vi "Run Bfr Tx - Sim Buffer Data.vi"(8 "error in (no error)":errorcluster, 11 "Tx Loop Data in":T1={"General Resources"={"Packet Name"="", "Packet ID"=0, "Local IP Address"="", "Local Port"=0, "Multicast"=FALSE, "Multicast IP Address"=0, "Header Info"=[], "Byte Order"=enum."big-endian, network order", "Channel Data Types"=[], "Duplex Packets"=refnum}, "Header Details"={"Packet Size"=0, "Protocol Revision"=0, "System Definition Version"=0, "Source Node Name"="", "Packet ID"=0, "Number of Channels"=0, "Static Header Size"=0, "Total Header Size"=0, "CustomHeaderLogic"={"CustomHeaderON"=FALSE, "CustomHeaderLogic"=""}}, "Buffer Resources"={"Data Buffer"=0, "Pointer Encoding"=enum."Direct Encoding", "Buffer Size"=0, "Buffer Size (I32)"=0, "Raw Buffer Data"=[], "Is Buffered"=FALSE, "External Buffer"=FALSE, "Prepend Header"=FALSE, "Valid Buffer"=FALSE}, "Runtime Resources"={"Connection ID"=refnum, "Transmit Option"=enum."Always", "Destination IP Address"=0, "Destination Port"=0, "Multicast IP Address"=0, "TTL"=0, "Multicast"=FALSE, "Port as Channel"=FALSE, "ExecutionConfig"={"Loop Period"=0, "RT Loop Period"=-2, "Untimed Period"=0, "Target Processor"=0, "Priority"=0, "Thread Management"=enum."Untimed (Default)"}}, "Echo Resources"={"Transmit Echo Option"=enum."PCL Reset", "Packet Count"=0.0, "Counter Increment"=0.0, "Transmit Values"=[]}, "Buffer Option Support"={"Buffer Option"=enum."Static Buffer", "Sim Option"=enum."No Simulation"}, "Channel Resources"={"Transmit Flag"=refnum, "Transmit Echo"=refnum, "Transmit Bytes"=refnum, "Port Channel"=refnum, "Buffer (External)"=refnum, "Buffer (Local)"=refnum, "Timestamp"=refnum}, "Debug Resources"={"Debug Mode"=FALSE, "Debug Log File"=refnum, "Packet Name"=""}} {"Buffer Resources"."Data Buffer" format="%016x"}) -> (0 "error out":errorcluster, 3 "Tx Loop Data out":T1={"General Resources"={"Packet Name"="", "Packet ID"=0, "Local IP Address"="", "Local Port"=0, "Multicast"=FALSE, "Multicast IP Address"=0, "Header Info"=[], "Byte Order"=enum."big-endian, network order", "Channel Data Types"=[], "Duplex Packets"=refnum}, "Header Details"={"Packet Size"=0, "Protocol Revision"=0, "System Definition Version"=0, "Source Node Name"="", "Packet ID"=0, "Number of Channels"=0, "Static Header Size"=0, "Total Header Size"=0, "CustomHeaderLogic"={"CustomHeaderON"=FALSE, "CustomHeaderLogic"=""}}, "Buffer Resources"={"Data Buffer"=0, "Pointer Encoding"=enum."Direct Encoding", "Buffer Size"=0, "Buffer Size (I32)"=0, "Raw Buffer Data"=[], "Is Buffered"=FALSE, "External Buffer"=FALSE, "Prepend Header"=FALSE, "Valid Buffer"=FALSE}, "Runtime Resources"={"Connection ID"=refnum, "Transmit Option"=enum."Always", "Destination IP Address"=0, "Destination Port"=0, "Multicast IP Address"=0, "TTL"=0, "Multicast"=FALSE, "Port as Channel"=FALSE, "ExecutionConfig"={"Loop Period"=0, "RT Loop Period"=-2, "Untimed Period"=0, "Target Processor"=0, "Priority"=0, "Thread Management"=enum."Untimed (Default)"}}, "Echo Resources"={"Transmit Echo Option"=enum."PCL Reset", "Packet Count"=0.0, "Counter Increment"=0.0, "Transmit Values"=[]}, "Buffer Option Support"={"Buffer Option"=enum."Static Buffer", "Sim Option"=enum."No Simulation"}, "Channel Resources"={"Transmit Flag"=refnum, "Transmit Echo"=refnum, "Transmit Bytes"=refnum, "Port Channel"=refnum, "Buffer (External)"=refnum, "Buffer (Local)"=refnum, "Timestamp"=refnum}, "Debug Resources"={"Debug Mode"=FALSE, "Debug Log File"=refnum, "Packet Name"=""}} {"Buffer Resources"."Data Buffer" format="%016x"})   [LabVIEW 2019, in "UDP-Custom-Device Engine.lvlib"]
uses:
  UDP-Custom-Device Engine.lvlib
  Types/Engine - Buffered Tx Loop Data.ctl
  Types/Engine - General Resources.ctl
  <vilib>/NI VeriStand/VeriStand Data/Typedefs/Typedefs.Data Types.ctl
  Shared/Types/Shared - Duplex Settings.ctl
  Shared/Types/Shared - Header Details.ctl
  Shared/Types/Shared - Custom Header.ctl
  Types/Engine - Buffer Resources.ctl
  Shared/Types/Shared - Pointer Encoding.ctl
  Types/Engine - Tx Runtime Resources.ctl
  Shared/Types/Shared - Transmit Flag Options.ctl
  Types/Engine - Execution Config.ctl
  Shared/Types/Shared - Thread Management.ctl
  Types/Engine - Tx Echo Resources.ctl
  Shared/Types/Shared - Transmit Echo Options.ctl
  Types/Engine - Buffered Tx Buffer Option Support.ctl
  Shared/Types/Shared - Transmit Buffer Options.ctl
  Shared/Types/Shared - Transmit Sim Options.ctl
  Types/Engine - Buffered Tx Channel Refs.ctl
  <vilib>/NI/NIVS Inline Async API/_Data Access Engine/Data Access Engine/Types/Read.DVR.ctl
  <vilib>/NI/NIVS Inline Async API/_Data Access Engine/Access Type Classes/Read/Read.lvclass
  <vilib>/NI/NIVS Inline Async API/_Data Access Engine/Data Access Engine/Types/Write.DVR.ctl
  <vilib>/NI/NIVS Inline Async API/_Data Access Engine/Access Type Classes/Write/Write.lvclass
  Types/Engine - Debug Resources.ctl
  <vilib>/NI/NIVS Inline Async API/_Data Access Engine/Access Type Classes/Read/Read.lvclass/Read.ctl
  <vilib>/NI VeriStand/VeriStand Data/Pointer Operations/Pointer.Write (String).vi
  <vilib>/NI VeriStand/VeriStand Data/Pointer Operations/Pointer.Write (1D U8).vi
  <vilib>/NI VeriStand/VeriStand Data/Pointer Operations/Pointer.Write (I32).vi
  <vilib>/NI VeriStand/VeriStand Data/Pointer Operations/Pointer.Write (U16).vi
  Transmit/Run Tx - Handle Transmit Option.vi
  Run Bfr Tx - Handle Transmit Size.vi
  Transmit/Run Tx - Handle Port Tx Check.vi
  <vilib>/NI/NIVS Inline Async API/_Data Access Engine/Data Access Engine/Methods/Data.Processes.Execute.vi
  <vilib>/NI/NIVS Inline Async API/_Data Access Engine/Data Access Engine/Methods/Read.Data.vi
  <vilib>/NI VeriStand/VeriStand Data/Type Conversion/Type Conversion.From Double.vi
  <vilib>/NI VeriStand/VeriStand Data/Type Conversion/Type Conversion.From Double (I32).vi
  <vilib>/NI/NIVS Inline Async API/_Data Access Engine/Access Type Classes/Read/Read.ProcessData.vi
  <vilib>/NI VeriStand/VeriStand Data/VeriStand Data.lvlib
  Shared/UDP-Custom-Device Shared.lvlib
  <vilib>/NI/NIVS Inline Async API/_Data Access Engine/Data Access Engine/Data Access Engine.lvclass
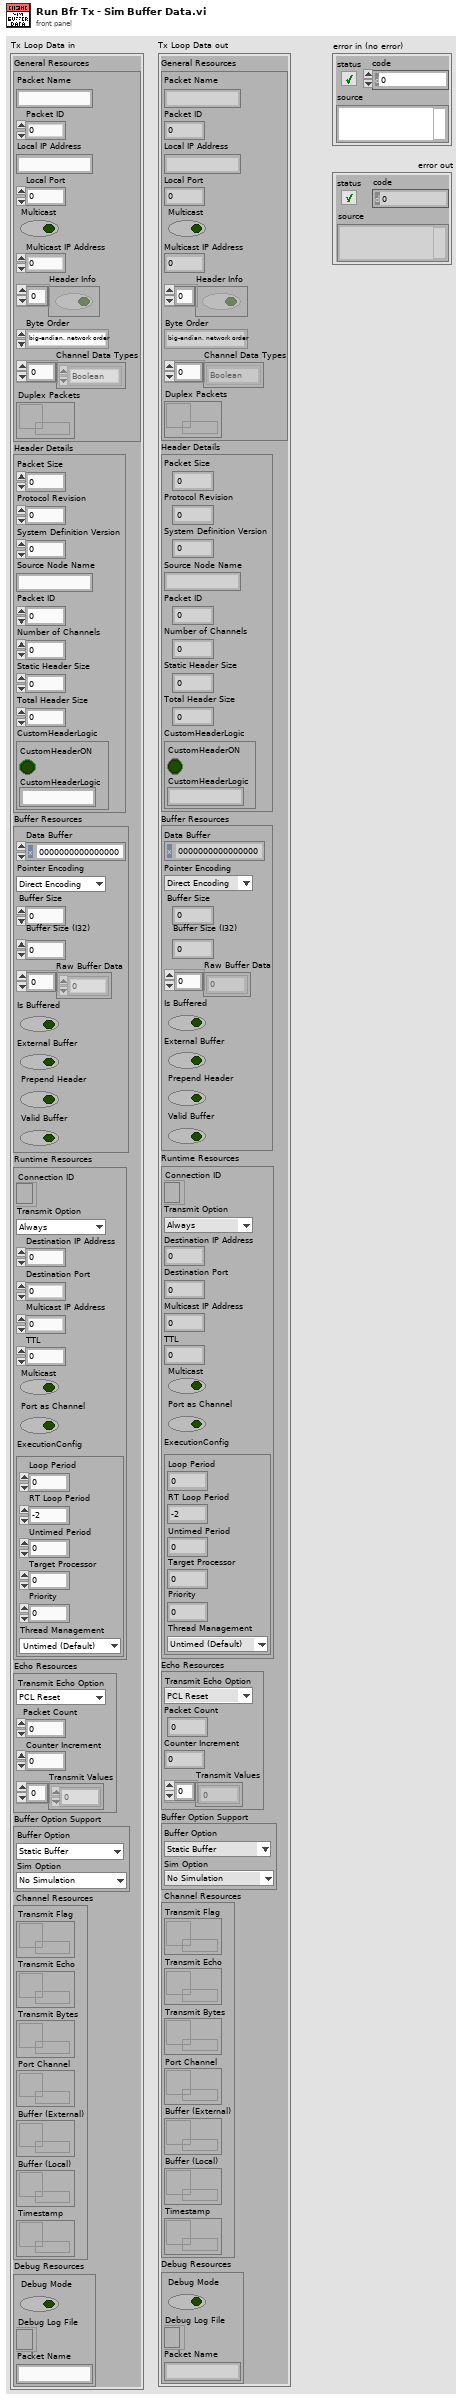
[diagram p1: front panel]
types:
  T1 = typedef "UDP-Custom-Device Engine.lvlib/Engine - Buffered Tx Loop Data.ctl" = cluster{"General Resources":T2, "Header Details":T4, "Buffer Resources":T6, "Runtime Resources":T8, "Echo Resources":T12, "Buffer Option Support":T14, "Channel Resources":T17, "Debug Resources":T20}
  T2 = typedef "UDP-Custom-Device Engine.lvlib/Engine - General Resources.ctl" = cluster{"Packet Name":string, "Packet ID":i32, "Local IP Address":string, "Local Port":i32, "Multicast":bool, "Multicast IP Address":u32, "Header Info":bool[], "Byte Order":enum16{"big-endian, network order", "native, host order", "little-endian"}, "Channel Data Types":T3[], "Duplex Packets":refnum<data-value>}
  T3 = typedef "VeriStand Data.lvlib/Typedefs.Data Types.ctl" = enum16{"Boolean", "Single", "Double", "I8", "I16", "I32", "I64", "U8", "U16", "U32", "U64"}
  T4 = typedef "UDP-Custom-Device Shared.lvlib/Shared - Header Details.ctl" = cluster{"Packet Size":u16, "Protocol Revision":u8, "System Definition Version":u64, "Source Node Name":string, "Packet ID":u32, "Number of Channels":u32, "Static Header Size":u16, "Total Header Size":u16, "CustomHeaderLogic":T5}
  T5 = typedef "UDP-Custom-Device Shared.lvlib/Shared - Custom Header.ctl" = cluster{"CustomHeaderON":bool, "CustomHeaderLogic":string}
  T6 = typedef "UDP-Custom-Device Engine.lvlib/Engine - Buffer Resources.ctl" = cluster{"Data Buffer":u64, "Pointer Encoding":T7, "Buffer Size":u64, "Buffer Size (I32)":i32, "Raw Buffer Data":u8[], "Is Buffered":bool, "External Buffer":bool, "Prepend Header":bool, "Valid Buffer":bool}
  T7 = typedef "UDP-Custom-Device Shared.lvlib/Shared - Pointer Encoding.ctl" = enum16{"Direct Encoding", "Conversion Encoding"}
  T8 = typedef "UDP-Custom-Device Engine.lvlib/Engine - Tx Runtime Resources.ctl" = cluster{"Connection ID":refnum<k16>, "Transmit Option":T9, "Destination IP Address":u32, "Destination Port":u16, "Multicast IP Address":u32, "TTL":u16, "Multicast":bool, "Port as Channel":bool, "ExecutionConfig":T10}
  T9 = typedef "UDP-Custom-Device Shared.lvlib/Shared - Transmit Flag Options.ctl" = enum16{"Always", "One-Shot", "Toggle"}
  T10 = typedef "UDP-Custom-Device Engine.lvlib/Engine - Execution Config.ctl" = cluster{"Loop Period":i64, "RT Loop Period":i64, "Untimed Period":u32, "Target Processor":i32, "Priority":i32, "Thread Management":T11}
  T11 = typedef "UDP-Custom-Device Shared.lvlib/Shared - Thread Management.ctl" = enum16{"Untimed (Default)", "Timed (High Priority)"}
  T12 = typedef "UDP-Custom-Device Engine.lvlib/Engine - Tx Echo Resources.ctl" = cluster{"Transmit Echo Option":T13, "Packet Count":dbl, "Counter Increment":dbl, "Transmit Values":dbl[]}
  T13 = typedef "UDP-Custom-Device Shared.lvlib/Shared - Transmit Echo Options.ctl" = enum16{"PCL Reset", "Counter", "Mirror"}
  T14 = typedef "UDP-Custom-Device Engine.lvlib/Engine - Buffered Tx Buffer Option Support.ctl" = cluster{"Buffer Option":T15, "Sim Option":T16}
  T15 = typedef "UDP-Custom-Device Shared.lvlib/Shared - Transmit Buffer Options.ctl" = enum16{"Static Buffer", "FIFO Buffer", "FIFO Buffer + Port"}
  T16 = typedef "UDP-Custom-Device Shared.lvlib/Shared - Transmit Sim Options.ctl" = enum16{"No Simulation", "Counter", "Full Buffer", "FIFO Test", "FIFO + Port Test"}
  T17 = typedef "UDP-Custom-Device Engine.lvlib/Engine - Buffered Tx Channel Refs.ctl" = cluster{"Transmit Flag":T18, "Transmit Echo":T19, "Transmit Bytes":T18, "Port Channel":T18, "Buffer (External)":T18, "Buffer (Local)":T19, "Timestamp":T18}
  T18 = typedef "Data Access Engine.lvlib/Data Access Engine.lvclass/Read.DVR.ctl" = refnum<data-value>
  T19 = typedef "Data Access Engine.lvlib/Data Access Engine.lvclass/Write.DVR.ctl" = refnum<data-value>
  T20 = typedef "UDP-Custom-Device Engine.lvlib/Engine - Debug Resources.ctl" = cluster{"Debug Mode":bool, "Debug Log File":refnum<file>, "Packet Name":string}
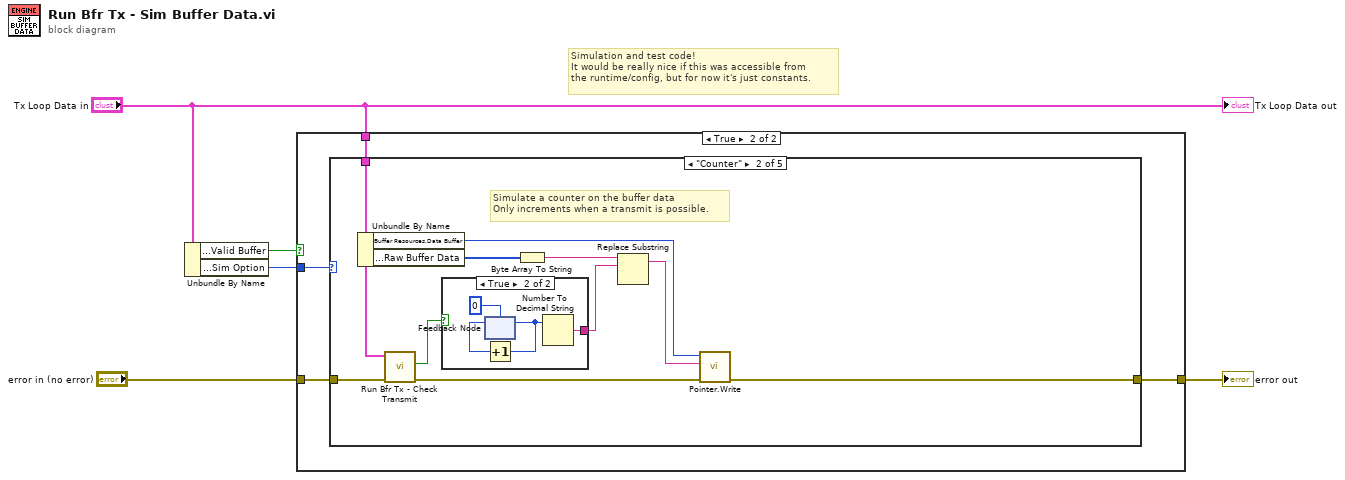
[diagram p0: block diagram]
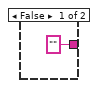
[diagram p4: hidden frame]
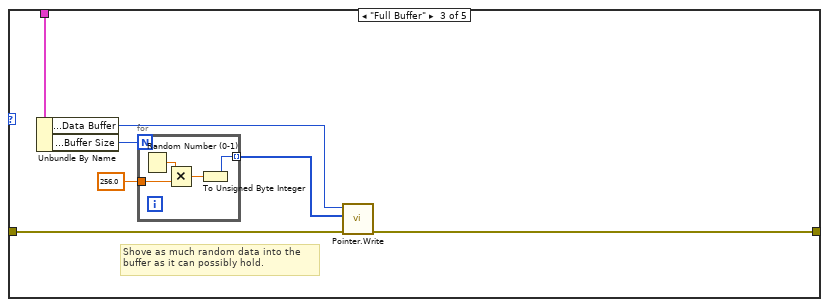
[diagram p5: hidden frame]
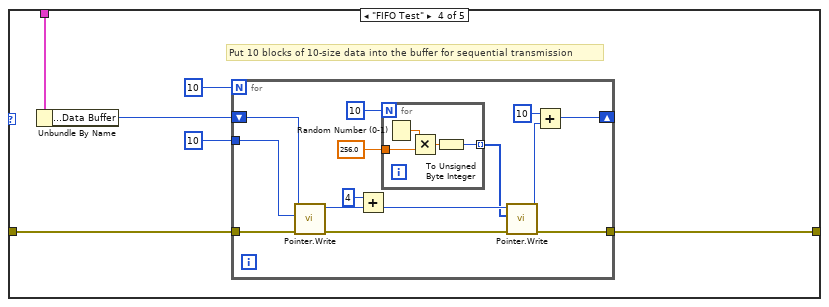
[diagram p6: hidden frame]
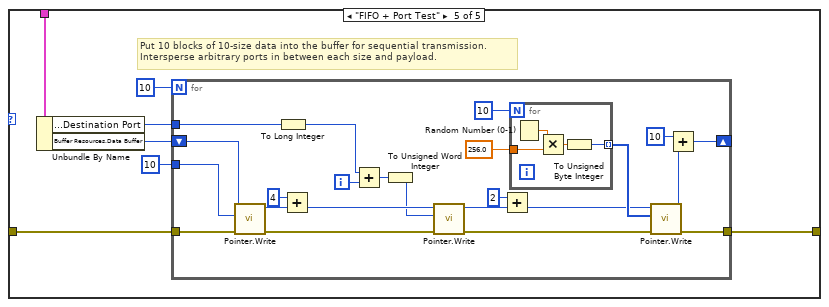
[diagram p7: hidden frame]
diagram:
  # "Simulation and test code!\nIt would be really nice if this was accessible from\nthe runtime/config, but for now it's just constants."
  n1 = Unbundle By Name("Tx Loop Data in") -> ("Buffer Resources.Valid Buffer"=w2:bool, "Buffer Option Support.Sim Option"=w1:T16)
  n2 = case shown="True" w2 {
    tunnel: "error in (no error)" -> [w6 w10]
    tunnel: [w6 w9] -> w4
    tunnel: "Tx Loop Data in" -> [_ w8]
    tunnel: w1 -> [_ w7]
    frame False {
    }
    frame True {
      n3 = case shown="\"Counter\"" w7 {
        tunnel: w8 -> [_ w15 w33 w43 w68]
        tunnel: w10 -> [w11 w14 w31 w39 w64]
        tunnel: [w11 w19 w30 w41 w66] -> w9
        frame "No Simulation", Default {
          # "No simulation data in normal\nbehavior."
        }
        frame "Counter" {
          # "Simulate a counter on the buffer data\nOnly increments when a transmit is possible."
          n4 = Unbundle By Name(w15) -> ("Buffer Resources.Data Buffer"=w21:u64, "Buffer Resources.Raw Buffer Data"=w17:u8[])
          n5 = call "Run Bfr Tx - Check Transmit.vi"("error in (no error)"=w14, "Tx Loop Data in"=w15) -> ("error out"=w13:errorcluster, "Transmit?"=w12:bool)  [unwired: 6 in, 2 out]
          n6 = case shown="True" w12 {
            tunnel: ["" w23] -> w20
            frame False {
            }
            frame True {
              n7 = feedback #1(0) -> (w25:i32)
              n8 = Increment(x=w25) -> (x+1=w24:i32)
              n9 = feedback-in #1(w24) -> ()
              n10 = Number To Decimal String(number=w24) -> (decimal integer string=w23:string)  [unwired: 1 in]
            }
          }
          n11 = Byte Array To String(unsigned byte array=w17) -> (string=w16:string)
          n12 = Replace Substring(4:w20, 5:w16) -> (1:w18:string)  [unwired: 2 in, 1 out]
          n13 = call-poly <vilib>:"Pointer.Write.vi"("error in (no error)"=w13, "string in"=w18, "pointer in"=w21) -> ("error out"=w19:errorcluster)  [unwired: 6 in, 2 out]
        }
        frame "Full Buffer" {
          # "Shove as much random data into the\nbuffer as it can possibly hold."
          n14 = Unbundle By Name(w33) -> ("Buffer Resources.Data Buffer"=w32:u64, "Buffer Resources.Buffer Size"=w29:u64)
          n15 = for {
            N: w29 -> [_]
            tunnel: [w34] -> w27 mode=indexing
            tunnel: 256.0 -> [w36]
            n16 = Random Number (0-1)() -> (number: 0 to 1=w37:dbl)
            n17 = Multiply(x=w37, y=w36) -> (x*y=w35:dbl)
            n18 = To Unsigned Byte Integer(number=w35) -> (unsigned 8bit integer=w34:u8)
          }
          n19 = call-poly <vilib>:"Pointer.Write.vi"("error in (no error)"=w31, "values"=w27, "pointer in"=w32) -> ("error out"=w30:errorcluster)  [unwired: 6 in, 2 out]
        }
        frame "FIFO Test" {
          # "Put 10 blocks of 10-size data into the buffer for sequential transmission"
          n20 = Unbundle By Name(w43) -> ("Buffer Resources.Data Buffer"=w42:u64)
          n21 = for {
            N: 10 -> [_]
            tunnel: [w57] -> w41
            tunnel: w39 -> [w55]
            tunnel: 10 -> [w53]
            shift-right: [w44] -> _
            shift-left: w42 -> [w56]
            n22 = call-poly <vilib>:"Pointer.Write.vi"("error in (no error)"=w55, "value"=w53, "pointer in"=w56) -> ("error out"=w54:errorcluster, "pointer out"=w51:u64)  [unwired: 6 in, 1 out]
            n23 = Add(x=u64 4, y=w51) -> (x+y=w50:u64)
            n24 = for {
              N: 10 -> [_]
              tunnel: [w58] -> w47 mode=indexing
              tunnel: 256.0 -> [w60]
              n25 = Random Number (0-1)() -> (number: 0 to 1=w61:dbl)
              n26 = Multiply(x=w61, y=w60) -> (x*y=w59:dbl)
              n27 = To Unsigned Byte Integer(number=w59) -> (unsigned 8bit integer=w58:u8)
            }
            n28 = call-poly <vilib>:"Pointer.Write.vi"("error in (no error)"=w54, "values"=w47, "pointer in"=w50) -> ("error out"=w57:errorcluster, "pointer out"=w45:u64)  [unwired: 6 in, 1 out]
            n29 = Add(x=u64 10, y=w45) -> (x+y=w44:u64)
          }
        }
        frame "FIFO + Port Test" {
          # "Put 10 blocks of 10-size data into the buffer for sequential transmission.\nIntersperse arbitrary ports in between each size and payload."
          n30 = Unbundle By Name(w68) -> ("Runtime Resources.Destination Port"=w62:u16, "Buffer Resources.Data Buffer"=w67:u64)
          n31 = for {
            N: 10 -> [_]
            tunnel: [w91] -> w66
            tunnel: w64 -> [w89]
            tunnel: 10 -> [w88]
            shift-right: [w80] -> _
            shift-left: w67 -> [w90]
            tunnel: w62 -> [w70]
            i -> [w72]
            n32 = call-poly <vilib>:"Pointer.Write.vi"("error in (no error)"=w89, "value"=w88, "pointer in"=w90) -> ("error out"=w78:errorcluster, "pointer out"=w86:u64)  [unwired: 6 in, 1 out]
            n33 = To Long Integer(number=w70) -> (32bit integer=w69:i32)
            n34 = Add(x=u64 4, y=w86) -> (x+y=w79:u64)
            n35 = Add(x=w69, y=w72) -> (x+y=w73:i32)
            n36 = To Unsigned Word Integer(number=w73) -> (unsigned 16bit integer=w71:u16)
            n37 = call-poly <vilib>:"Pointer.Write.vi"("error in (no error)"=w78, "value"=w71, "pointer in"=w79) -> ("error out"=w77:errorcluster, "pointer out"=w75:u64)  [unwired: 6 in, 1 out]
            n38 = Add(x=u64 2, y=w75) -> (x+y=w74:u64)
            n39 = for {
              N: 10 -> [_]
              tunnel: [w92] -> w83 mode=indexing
              tunnel: 256.0 -> [w94]
              n40 = Random Number (0-1)() -> (number: 0 to 1=w95:dbl)
              n41 = Multiply(x=w95, y=w94) -> (x*y=w93:dbl)
              n42 = To Unsigned Byte Integer(number=w93) -> (unsigned 8bit integer=w92:u8)
            }
            n43 = call-poly <vilib>:"Pointer.Write.vi"("error in (no error)"=w77, "values"=w83, "pointer in"=w74) -> ("error out"=w91:errorcluster, "pointer out"=w81:u64)  [unwired: 6 in, 1 out]
            n44 = Add(x=u64 10, y=w81) -> (x+y=w80:u64)
          }
        }
      }
    }
  }
  "error out" <- w4
  "Tx Loop Data out" <- "Tx Loop Data in"
